vi "Box Size Filter (SubVI).vi"(0 "Particle Statistics":T1, 1 "Box Side":cluster{"Low":u32, "High":u32}={"Low"=15, "High"=255}, 2 "Box W + L":cluster{"Low":u32, "High":u32}={"Low"=15, "High"=255}, 3 "Area":cluster{"Low":u32, "High":u32}={"Low"=15, "High"=255}, 5 "Input Valid":bool, 9 "EOI In":bool) -> (4 "Bounding Box":u64, 8 "Data Valid":bool, 15 "EOI Out":bool)   [LabVIEW 2015]
uses:
  <vilib>/visionFPGA/Analysis/ParticleAnalysisReport/SubVIs/WithoutHoles/Particle Statistics without Holes.ctl
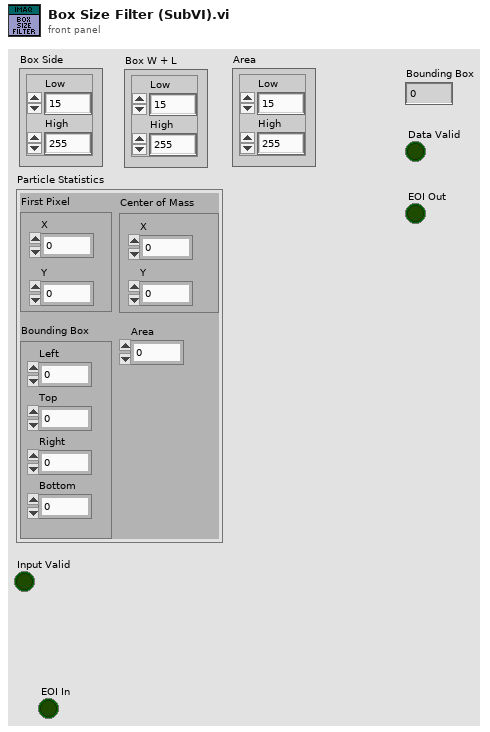
[diagram p1: front panel]
types:
  T1 = typedef "Particle Statistics without Holes.ctl" = cluster{"First Pixel":cluster{"X":i32, "Y":i32}, "Bounding Box":cluster{"Left":i32, "Top":i32, "Right":i32, "Bottom":i32}, "Center of Mass":cluster{"X":fxp<+/-,48,32>, "Y":fxp<+/-,48,32>}, "Area":u32}
  T2 = cluster{"Left":i32, "Top":i32, "Right":i32, "Bottom":i32}
  T3 = cluster{"Left":i16, "Top":i16, "Right":i16, "Bottom":i16}
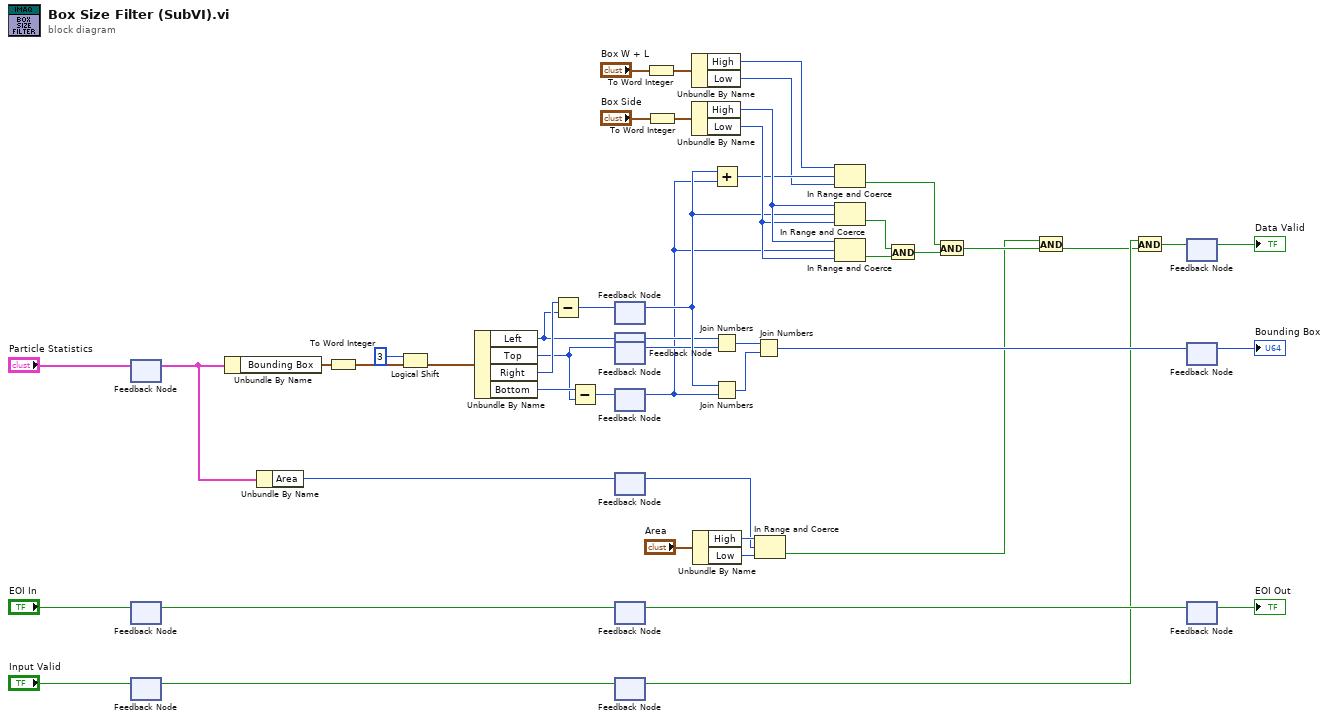
[diagram p0: block diagram]
diagram:
  n1 = feedback-in #1("Particle Statistics") -> ()
  n2 = feedback #1() -> (w7:T1)  [unwired: 1 in]
  n3 = feedback-in #2("EOI In") -> ()
  n4 = feedback #2() -> (w36:bool)  [unwired: 1 in]
  n5 = feedback-in #3("Input Valid") -> ()
  n6 = feedback #3() -> (w35:bool)  [unwired: 1 in]
  n7 = Unbundle By Name(w7) -> ("Bounding Box"=w39:T2)
  n8 = Unbundle By Name(w7) -> ("Area"=w3:u32)
  n9 = To Word Integer(number=w39) -> (16bit integer=w42:T3)
  n10 = Logical Shift(y=i16 3, x=w42) -> (x << y=w32:T3)
  n11 = Unbundle By Name(w32) -> ("Left"=w34:i16, "Top"=w33:i16, "Right"=w40:i16, "Bottom"=w41:i16)
  n12 = Subtract(x=w40, y=w34) -> (x-y=w24:i16)
  n13 = Subtract(x=w41, y=w33) -> (x-y=w23:i16)
  n14 = feedback-in #4(w24) -> ()
  n15 = feedback #4() -> (w22:i16)  [unwired: 1 in]
  n16 = feedback-in #5(w34) -> ()
  n17 = feedback #5() -> (w20:i16)  [unwired: 1 in]
  n18 = feedback-in #6(w33) -> ()
  n19 = feedback #6() -> (w21:i16)  [unwired: 1 in]
  n20 = feedback-in #7(w23) -> ()
  n21 = feedback #7() -> (w19:i16)  [unwired: 1 in]
  n22 = feedback-in #8(w3) -> ()
  n23 = feedback #8() -> (w1:u32)  [unwired: 1 in]
  n24 = feedback-in #9(w36) -> ()
  n25 = feedback #9() -> (w18:bool)  [unwired: 1 in]
  n26 = feedback-in #10(w35) -> ()
  n27 = feedback #10() -> (w16:bool)  [unwired: 1 in]
  n28 = To Word Integer(number="Box W + L") -> (16bit integer=w14:cluster{"Low":i16, "High":i16})
  n29 = To Word Integer(number="Box Side") -> (16bit integer=w30:cluster{"Low":i16, "High":i16})
  n30 = Unbundle By Name(w14) -> ("High"=w11:i16, "Low"=w10:i16)
  n31 = Unbundle By Name(w30) -> ("High"=w29:i16, "Low"=w28:i16)
  n32 = Unbundle By Name("Area") -> ("High"=w5:u32, "Low"=w4:u32)
  n33 = Add(x=w22, y=w19) -> (x+y=w12:i16)
  n34 = Join Numbers(hi=w20, lo=w21) -> ((hi.lo)=w43:u32)
  n35 = Join Numbers(hi=w22, lo=w19) -> ((hi.lo)=w44:u32)
  n36 = Join Numbers(hi=w43, lo=w44) -> ((hi.lo)=w45:u64)
  n37 = In Range and Coerce(upper limit=w5, x=w1, lower limit=w4) -> (In Range?=w2:bool)  [unwired: 1 out]
  n38 = In Range and Coerce(upper limit=w11, x=w12, lower limit=w10) -> (In Range?=w15:bool)  [unwired: 1 out]
  n39 = In Range and Coerce(upper limit=w29, x=w22, lower limit=w28) -> (In Range?=w26:bool)  [unwired: 1 out]
  n40 = In Range and Coerce(upper limit=w29, x=w19, lower limit=w28) -> (In Range?=w25:bool)  [unwired: 1 out]
  n41 = And(x=w26, y=w25) -> (x .and. y?=w27:bool)
  n42 = And(x=w15, y=w27) -> (x .and. y?=w49:bool)
  n43 = And(x=w2, y=w49) -> (x .and. y?=w8:bool)
  n44 = And(x=w16, y=w8) -> (x .and. y?=w17:bool)
  n45 = feedback-in #11(w17) -> ()
  n46 = feedback #11() -> (→"Data Valid":bool)  [unwired: 1 in]
  n47 = feedback-in #12(w45) -> ()
  n48 = feedback #12() -> (→"Bounding Box":u64)  [unwired: 1 in]
  n49 = feedback #13() -> (→"EOI Out":bool)  [unwired: 1 in]
  n50 = feedback-in #13(w18) -> ()
